vi "VI Tree.vi"   [LabVIEW 2012, in "Agilent 34970.lvlib"]
doc: "This is the LV instrument driver for the HP 34970A Data Acquisition / Switch Unit. The VI Tree shows all of the User-Callable VIs in the instrument driver in an organized table. \n\nHewlett-Packard\nHP 34970A Data Acquisition / Switch Unit\n\nThis instrument driver's revision number is \"REV 1.0, 02/98, LV 4.1\" and is compatable with instrument firmware revision: \"0.87\"\n\nAuthor: Paul Davis\nCompany: VI Technology\nPhone: 512.327.3348\nEmail: paul.davis@vi-tech.com\nRelease date: February 1998\n\nOriginally developed in LabVIEW Version: 4.1"
uses:
  <instrlib>/Agilent 34970/Agilent 34970.lvlib
panel:
  # "(c) 2005-2010 National Instruments.  ALL RIGHTS RESERVED."
  # "SEE DIAGRAM\nFOR VI TREE."
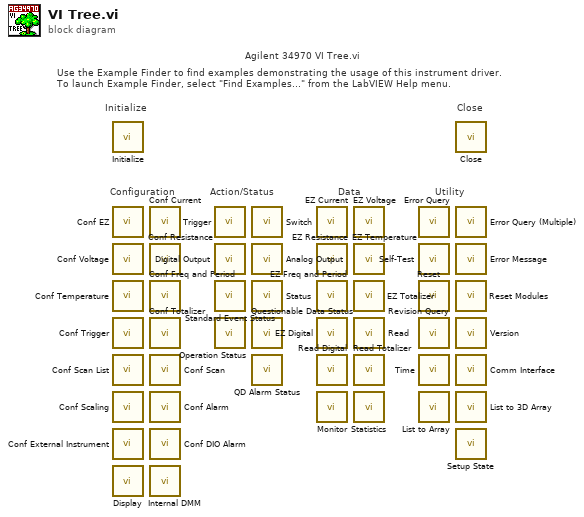
[diagram p0: block diagram]
diagram:
  # "Agilent 34970 VI Tree.vi"
  # "Use the Example Finder to find examples demonstrating the usage of this instrument driver.\nTo launch Example Finder, select \"Find Examples...\" from the LabVIEW Help menu."
  # "Configuration"
  # "Utility"
  # "Data"
  # "Action/Status"
  # "Close"
  # "Initialize"
  n1 = call <instrlib>:"Initialize.vi"() -> ()  [unwired: 14 in, 2 out]
  n2 = call <instrlib>:"Conf EZ.vi"() -> ()  [unwired: 13 in, 3 out]
  n3 = call <instrlib>:"Conf Voltage.vi"() -> ()  [unwired: 13 in, 3 out]
  n4 = call <instrlib>:"Conf Temperature.vi"() -> ()  [unwired: 13 in, 3 out]
  n5 = call <instrlib>:"Conf Trigger.vi"() -> ()  [unwired: 13 in, 3 out]
  n6 = call <instrlib>:"Conf Scan List.vi"() -> ()  [unwired: 9 in, 3 out]
  n7 = call <instrlib>:"Conf Scaling.vi"() -> ()  [unwired: 13 in, 3 out]
  n8 = call <instrlib>:"Conf External Instrument.vi"() -> ()  [unwired: 9 in, 3 out]
  n9 = call <instrlib>:"Display.vi"() -> ()  [unwired: 8 in, 4 out]
  n10 = call <instrlib>:"Conf Current.vi"() -> ()  [unwired: 13 in, 3 out]
  n11 = call <instrlib>:"Conf Resistance.vi"() -> ()  [unwired: 13 in, 3 out]
  n12 = call <instrlib>:"Conf Freq and Period.vi"() -> ()  [unwired: 13 in, 3 out]
  n13 = call <instrlib>:"Conf Totalizer.vi"() -> ()  [unwired: 13 in, 3 out]
  n14 = call <instrlib>:"Conf Scan.vi"() -> ()  [unwired: 13 in, 3 out]
  n15 = call <instrlib>:"Conf Alarm.vi"() -> ()  [unwired: 17 in, 3 out]
  n16 = call <instrlib>:"Conf DIO Alarm.vi"() -> ()  [unwired: 17 in, 3 out]
  n17 = call <instrlib>:"Internal DMM.vi"() -> ()  [unwired: 9 in, 3 out]
  n18 = call <instrlib>:"Trigger.vi"() -> ()  [unwired: 10 in, 2 out]
  n19 = call <instrlib>:"Digital Output.vi"() -> ()  [unwired: 9 in, 3 out]
  n20 = call <instrlib>:"Standard Event Status.vi"() -> ()  [unwired: 9 in, 3 out]
  n21 = call <instrlib>:"Operation Status.vi"() -> ()  [unwired: 9 in, 3 out]
  n22 = call <instrlib>:"Switch.vi"() -> ()  [unwired: 9 in, 3 out]
  n23 = call <instrlib>:"Analog Output.vi"() -> ()  [unwired: 9 in, 3 out]
  n24 = call <instrlib>:"Status.vi"() -> ()  [unwired: 9 in, 3 out]
  n25 = call <instrlib>:"Questionable Data Status.vi"() -> ()  [unwired: 9 in, 3 out]
  n26 = call <instrlib>:"QD Alarm Status.vi"() -> ()  [unwired: 8 in, 4 out]
  n27 = call <instrlib>:"EZ Current.vi"() -> ()  [unwired: 9 in, 3 out]
  n28 = call <instrlib>:"EZ Resistance.vi"() -> ()  [unwired: 9 in, 3 out]
  n29 = call <instrlib>:"EZ Freq and Period.vi"() -> ()  [unwired: 9 in, 3 out]
  n30 = call <instrlib>:"EZ Digital.vi"() -> ()  [unwired: 9 in, 3 out]
  n31 = call <instrlib>:"Read Digital.vi"() -> ()  [unwired: 9 in, 3 out]
  n32 = call <instrlib>:"Monitor.vi"() -> ()  [unwired: 7 in, 5 out]
  n33 = call <instrlib>:"EZ Voltage.vi"() -> ()  [unwired: 9 in, 3 out]
  n34 = call <instrlib>:"EZ Temperature.vi"() -> ()  [unwired: 13 in, 3 out]
  n35 = call <instrlib>:"EZ Totalizer.vi"() -> ()  [unwired: 9 in, 3 out]
  n36 = call <instrlib>:"Read.vi"() -> ()  [unwired: 8 in, 4 out]
  n37 = call <instrlib>:"Read Totalizer.vi"() -> ()  [unwired: 9 in, 3 out]
  n38 = call <instrlib>:"Statistics.vi"() -> ()  [unwired: 8 in, 4 out]
  n39 = call <instrlib>:"Error Query.vi"() -> ()  [unwired: 12 in, 4 out]
  n40 = call <instrlib>:"Self-Test.vi"() -> ()  [unwired: 12 in, 4 out]
  n41 = call <instrlib>:"Reset.vi"() -> ()  [unwired: 14 in, 2 out]
  n42 = call <instrlib>:"Revision Query.vi"() -> ()  [unwired: 8 in, 4 out]
  n43 = call <instrlib>:"Time.vi"() -> ()  [unwired: 9 in, 3 out]
  n44 = call <instrlib>:"List to Array.vi"() -> ()  [unwired: 10 in, 2 out]
  n45 = call <instrlib>:"Close.vi"() -> ()  [unwired: 15 in, 1 out]
  n46 = call <instrlib>:"Error Query (Multiple).vi"() -> ()  [unwired: 12 in, 4 out]
  n47 = call <instrlib>:"Error Message.vi"() -> ()  [unwired: 11 in, 5 out]
  n48 = call <instrlib>:"Reset Modules.vi"() -> ()  [unwired: 10 in, 2 out]
  n49 = call <instrlib>:"Version.vi"() -> ()  [unwired: 7 in, 9 out]
  n50 = call <instrlib>:"Comm Interface.vi"() -> ()  [unwired: 9 in, 3 out]
  n51 = call <instrlib>:"List to 3D Array.vi"() -> ()  [unwired: 11 in, 1 out]
  n52 = call <instrlib>:"Setup State.vi"() -> ()  [unwired: 10 in, 2 out]
